vi "Constructor_RQMHStartup.vi"(7 "Autoshutdown? (T)":bool, 8 "error in (no error)":errorcluster, 10 "StartupParams":variant, 11 "Already Running?":bool) -> (0 "error out":errorcluster, 3 "JQMHStartup out":refnum<class "RQMHStartup.lvclass">)   [LabVIEW 2024, in "RQMHStartup.lvclass"]
uses:
  RQMHStartup.lvclass
  Shared/Died.ctl
  Message.ctl
  Command.ctl
  RQMHStartup.lvclass/RQMHStartup.ctl
  Shared/RQMHShared.lvlib
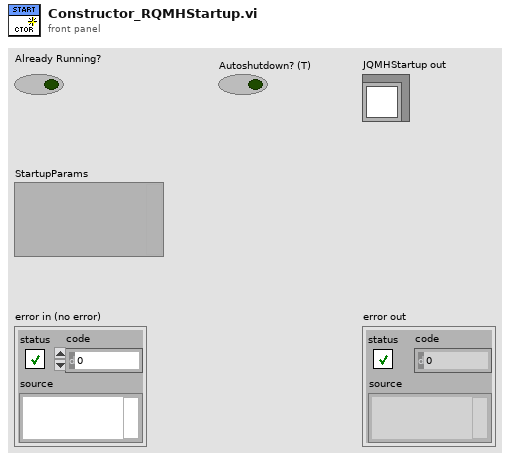
[diagram p1: front panel]
types:
  T1 = typedef "RQMHStartup.lvclass/Message.ctl" = cluster{"Command":T2, "Data":variant}
  T2 = typedef "RQMHStartup.lvclass/Command.ctl" = enum16{"Default", "No Override", "Error", "ACK Created", "ACK Mod Reg", "ACK Caller Reg"}
  T3 = typedef "RQMHShared.lvlib/Died.ctl" = bool
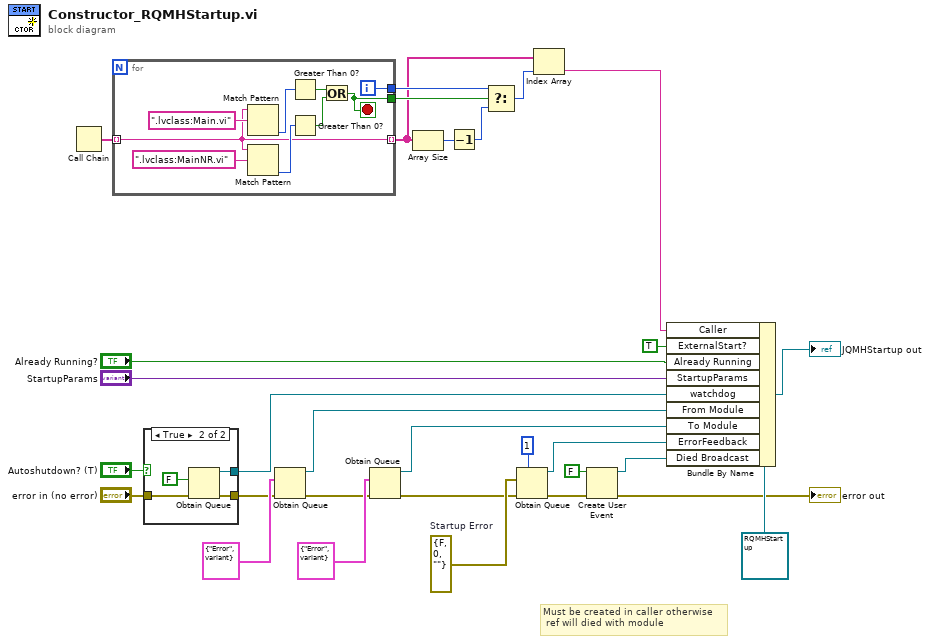
[diagram p0: block diagram]
diagram:
  w19 = errorcluster {"status"=FALSE, "code"=0, "source"=""}  # Startup Error
  # "Must be created in caller otherwise\n ref will died with module"
  n1 = Call Chain() -> (call chain=w8:string[])
  n2 = for {
    tunnel: w8 -> [w33] mode=indexing
    tunnel: [w33] -> w3 mode=indexing
    tunnel: [w32] -> w6
    tunnel: [w31] -> w7
    i -> [w32]
    stop <- w31 stop-if-true
    n3 = Match Pattern(string=w33, regular expression=".lvclass:Main.vi") -> (offset past match=w38:i32)  [unwired: 1 in, 3 out]
    n4 = Match Pattern(string=w33, regular expression=".lvclass:MainNR.vi") -> (offset past match=w37:i32)  [unwired: 1 in, 3 out]
    n5 = Greater Than 0?(x=w38) -> (x > 0?=w35:bool)
    n6 = Greater Than 0?(x=w37) -> (x > 0?=w34:bool)
    n7 = Or(x=w35, y=w34) -> (x .or. y?=w31:bool)
  }
  n8 = case shown="True" "Autoshutdown? (T)" {
    tunnel: [_ w43] -> w15
    tunnel: "error in (no error)" -> [w40 w42]
    tunnel: [w40 w41] -> w24
    frame False {
    }
    frame True {
      n9 = Obtain Queue(element data type=FALSE, error in (no error)=w42) -> (queue out=w43:refnum<queue>, error out=w41:errorcluster)  [unwired: 3 in, 1 out]
    }
  }
  n10 = Obtain Queue(element data type=T1 {"Command"=enum."Error", "Data"=variant} ("Handshake"), error in (no error)=w24) -> (queue out=w16:refnum<queue>, error out=w13:errorcluster)  [unwired: 3 in, 1 out]
  n11 = Obtain Queue(element data type=T1 {"Command"=enum."Error", "Data"=variant} ("Handshake"), error in (no error)=w13) -> (queue out=w11:refnum<queue>, error out=w12:errorcluster)  [unwired: 3 in, 1 out]
  n12 = Array Size(array=w3) -> (size(s)=w5:i32)
  n13 = Decrement(x=w5) -> (x-1=w4:i32)
  n14 = Select(t=w6, s=w7, f=w4) -> (s? t:f=w2:i32)
  n15 = Obtain Queue(max queue size (-1, unlimited)=1, element data type=w19, error in (no error)=w12) -> (queue out=w18:refnum<queue>, error out=w20:errorcluster)  [unwired: 2 in, 1 out]
  n16 = Index Array(array=w3, index=w2) -> (element=w1:string)
  n17 = Create User Event(user event datatype=T3 FALSE ("Died"), error in=w20) -> (user event=w23:refnum<user-event>, error out=→"error out":errorcluster)
  n18 = Bundle By Name(cluster=refnum<class "RQMHStartup.lvclass"> refnum ("JQMHStartup in"), "Caller"=w1, "ExternalStart?"=TRUE, "Already Running"="Already Running?", "StartupParams"="StartupParams", "watchdog"=w15, "From Module"=w16, "To Module"=w11, "ErrorFeedback"=w18, "Died Broadcast"=w23) -> (→"JQMHStartup out":refnum<class "RQMHStartup.lvclass">)
